vi "Clock.vi"(9 "Pulse counter in":u64, 10 "FPGA cycles per clock cycle":u64, 11 "Cycle counter in":u64) -> (1 "Pulse counter out":u64, 2 "Clock out":bool, 3 "Cycle counter out":u64)   [LabVIEW 2012]
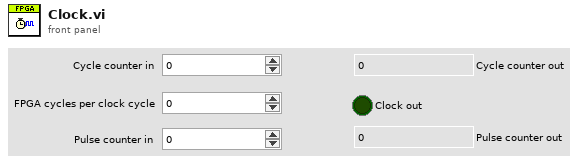
[diagram p1: front panel]
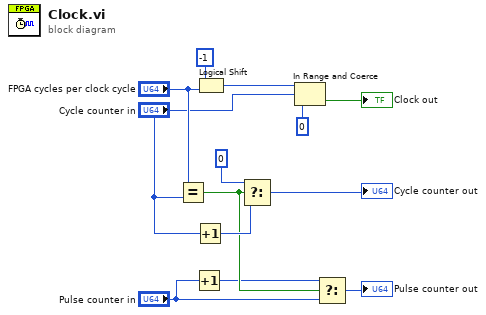
[diagram p0: block diagram]
diagram:
  n1 = Equal?(x="FPGA cycles per clock cycle", y="Cycle counter in") -> (x = y?=w4:bool)
  n2 = Increment(x="Pulse counter in") -> (x+1=w3:u64)
  n3 = Increment(x="Cycle counter in") -> (x+1=w7:u64)
  n4 = Logical Shift(y=i8 -1, x="FPGA cycles per clock cycle") -> (x << y=w11:u64)
  n5 = Select(t=u64 0, s=w4, f=w7) -> (s? t:f=→"Cycle counter out":u64)
  n6 = In Range and Coerce(upper limit=w11, x="Cycle counter in", lower limit=u64 0) -> (In Range?=→"Clock out":bool)  [unwired: 1 out]
  n7 = Select(t=w3, s=w4, f="Pulse counter in") -> (s? t:f=→"Pulse counter out":u64)
